vi "CloseAllVIRefs.vi"(1 "SlideInfo":T1[](array[typedef]), 2 "Scene.Object IN":refnum<vi>) -> ()   [LabVIEW 2010]
uses:
  SlideTypeDef.ctl
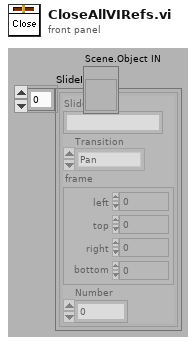
[diagram p1: front panel]
types:
  T1 = typedef "SlideTypeDef.ctl" = cluster{"Slide path":string, "Transition":enum16{"Pan", "Zoom-pan-zoom", "Zoom-wait-Zoom"}, "frame":cluster{"left":i16, "top":i16, "right":i16, "bottom":i16}, "Number":i32}
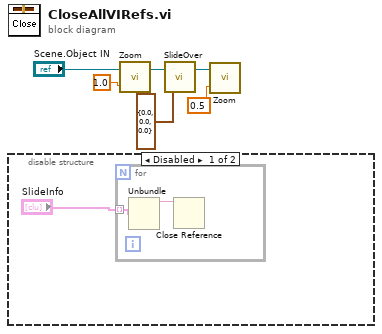
[diagram p0: block diagram]
diagram:
  n1 = disable-structure shown="Disabled" {
    frame Disabled {
      n2 = for {
        tunnel: "SlideInfo" -> [w9] mode=indexing
        n3 = Unbundle(w9) -> ("Slide path"=w8:string)  [unwired: 3 out]
        n4 = Close Reference(reference=w8) -> ()  [unwired: 1 in, 1 out]
      }
    }
    frame Enabled {
    }
  }
  n5 = call "Zoom.vi"("Final Zoom"=sgl 1.0, "Scene.Object IN"="Scene.Object IN") -> ("Scene.Object Out"=w6:refnum<vi>)  [unwired: 1 in]
  n6 = call "SlideOver.vi"("Location"=cluster{"X":sgl, "Y":sgl, "Z":sgl} {"X"=0.0, "Y"=0.0, "Z"=0.0}, "Scene.Object IN"=w6) -> ("Scene.Object Out"=w4:refnum<vi>)  [unwired: 1 in]
  n7 = call "Zoom.vi"("Final Zoom"=sgl 0.5, "Scene.Object IN"=w4) -> ()  [unwired: 1 in, 1 out]
